vi "Heartbeat check.vi"(4 "error in":errorcluster, 7 "CANopen in":refnum<class "CANopen.lvclass">) -> (0 "error out":errorcluster, 3 "CANopen out":refnum<class "CANopen.lvclass">)   [LabVIEW 2017, in "canopen.lvlib" / "CANopen.lvclass"]
doc: "Checks for watchdogs alarm in the heartbeat table. If a watchdog has elapsed, the error cluster is set accordingly."
uses:
  CANopen.lvclass
  CANopen.lvclass/CANopen.ctl
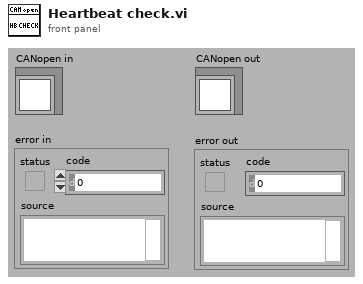
[diagram p1: front panel]
types:
  T1 = cluster{"Node ID":u8, "Period":dbl, "Set value":i16, "Value":i16}[]
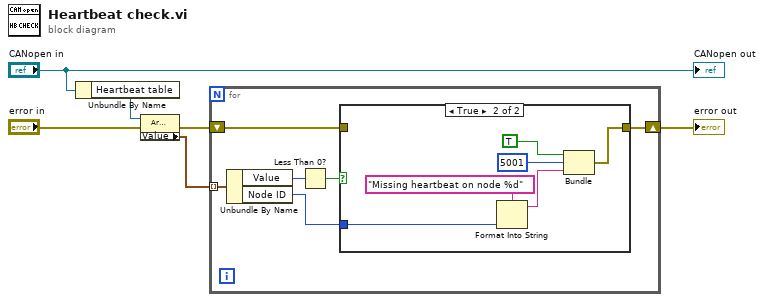
[diagram p0: block diagram]
diagram:
  n1 = Unbundle By Name("CANopen in") -> ("Heartbeat table"=w6:refnum<vi>)
  n2 = property class="Arr (strict)"(reference=w6, error in="error in") -> (error out=w2:errorcluster, "Value"=w4:T1)  [unwired: 1 out]
  n3 = for {
    tunnel: w4 -> [w12] mode=indexing
    shift-right: [w8] -> w1
    shift-left: w2 -> [w9]
    n4 = Unbundle By Name(w12) -> ("Value"=w11:i16, "Node ID"=w7:u8)
    n5 = Less Than 0?(x=w11) -> (x < 0?=w10:bool)
    n6 = case shown="True" w10 {
      tunnel: w9 -> [w13 _]
      tunnel: [w13 w17] -> w8
      tunnel: w7 -> [_ w15]
      frame False {
      }
      frame True {
        n7 = Format Into String(format string="Missing heartbeat on node %d" ("source"), w15) -> (resulting string=w14:string)  [unwired: 2 in, 1 out]
        n8 = Bundle("status"=TRUE, "code"=5001, w14) -> (w17:cluster{"status":bool, "code":i32, string})  [unwired: 1 out]
      }
    }
  }
  "error out" <- w1
  "CANopen out" <- "CANopen in"
